vi "Test Process within Nested App Log Info Message.vi"(8 "error in (no error)":errorcluster, 11 "Test Case In":refnum<class "Logger Test.lvclass">) -> (0 "error out":errorcluster, 3 "Test Case Out":refnum<class "Logger Test.lvclass">)   [LabVIEW 2020, in "Logger Test.lvclass"]
uses:
  Logger Test.lvclass
  C:/Program Files (x86)/National Instruments/LabVIEW 2020/vi.lib/Astemes/LUnit/Test Case.lvclass
  source/Framework Test Suite/Mock Log Handler/Mock Log Handler.lvclass
  C:/Git/astemes-triarc-framework/source/Framework/Logging/Logging.lvclass
  source/Framework Test Suite/Mock Process/Mock Process.lvclass
  C:/Git/astemes-triarc-framework/source/Framework/Process/Process.lvclass
  source/Framework/Application/Application.lvclass
  source/Framework/Process/Process.lvclass/Process.ctl
  source/Framework/Application/Application.lvclass/Application.ctl
  <vilib>/Astemes/LUnit/Test Case.lvclass/Test Case.ctl
  <vilib>/Astemes/LUnit/LUnit Assertion Result.lvclass/LUnit Assertion Result.ctl
  <vilib>/Astemes/LUnit/LUnit Test Case Result.lvclass/LUnit Test Case Result.ctl
  <vilib>/Astemes/LUnit/LUnit Method Result.lvclass/LUnit Method Result.ctl
  9c4a66fc-af29-4a58-8a71-606aefca4567.vi
  ff660fc9-a87e-4241-bf4f-74109907e361.vi
  4b535133-13cd-4873-93c4-223ebd3dba1f.vi
  source/Framework/Application/Private/Add Process to Map.vi
  source/Framework/Application/Private/Start Idle Processes if Running.vi
  source/Framework/Application/Private/Throw Error If Process Already in App.vi
  source/Framework/Process/Protected/Messaging/Enqueue Message.vi
  source/Framework/Process/Public/Lifecycle/Get Lifecycle State.vi
  source/Framework/Process/Protected/SubVIs/Set Context.vi
  source/Framework/Process/Private/SubVIs/Wait for finish.vi
  source/Framework/Process/Private/SubVIs/Set Lifecycle State.vi
  <vilib>/Astemes/LUnit/Palette/Pass.vi
  <vilib>/Astemes/LUnit/Palette/Fail.vi
  <vilib>/Astemes/LUnit/Compare Variants.vi
  <vilib>/Astemes/LUnit/Describe Comparison.vi
  <vilib>/Astemes/LUnit/Set Assertion Type.vi
  source/Framework/Application/Public/Get Process.vi
  source/Framework/Process/Private/SubVIs/Handle Debug Data.vi
  source/Framework/Process/Public/Lifecycle/Leave Process Loop.vi
  <vilib>/Astemes/LUnit/Add test result.vi
  <vilib>/Astemes/LUnit/LUnit Write Passed.vi
  <vilib>/Astemes/LUnit/LUnit Write Message.vi
  <vilib>/Astemes/LUnit/LUnit Write Description.vi
  <vilib>/Astemes/LUnit/Variant to string.vi
  <vilib>/Astemes/LUnit/LUnit Write Assertion Type.vi
  source/Framework/Application/Private/Retrieve Process from App.vi
  source/Framework/Application/Private/Parse Process Name.vi
  source/Framework/Application/Private/Get Process from Map.vi
  source/Framework/Logging/Log Debug.vi
  <vilib>/AdvancedString/1D String Array to Delimited String.vi
  <vilib>/Utility/High Resolution Relative Seconds.vi
  <vilib>/Astemes/LUnit/LUnit Record Assertion Result.vi
  source/Framework/Process/Protected/Messaging/Request Message.vi
  <vilib>/AdvancedString/Delimited String to 1D String Array.vi
  <vilib>/Astemes/LUnit/LUnit Aggregate Assertion Results.vi
  source/Framework/Process/Private/SubVIs/Enqueue Request Message.vi
  <vilib>/Astemes/LUnit/Assertion Result/LUnit Read Status.vi
  <vilib>/Astemes/LUnit/LUnit Read Message.vi
  <vilib>/Astemes/LUnit/LUnit Read Description.vi
  <vilib>/Astemes/LUnit/Method Result/LUnit Merge Status.vi
  <vilib>/Astemes/LUnit/LUnit Concatenate result strings.vi
  <vilib>/Utility/error.llb/Error Cluster From Error Code.vi
  source/Framework/Process/Public/Read Name.vi
  source/Framework/Process/Private/SubVIs/Wait for Response Message.vi
  <vilib>/Utility/Data Type/Get Type Information.vi
  <vilib>/Utility/LVClass/Get LV Class Name.vi
  source/Framework/Process/Process.lvclass
  <vilib>/Astemes/LUnit/LUnit Assertion Result.lvclass
  source/Framework/Logging/Logging.lvclass
  source/Framework Test Suite/Support/Test Support.lvlib
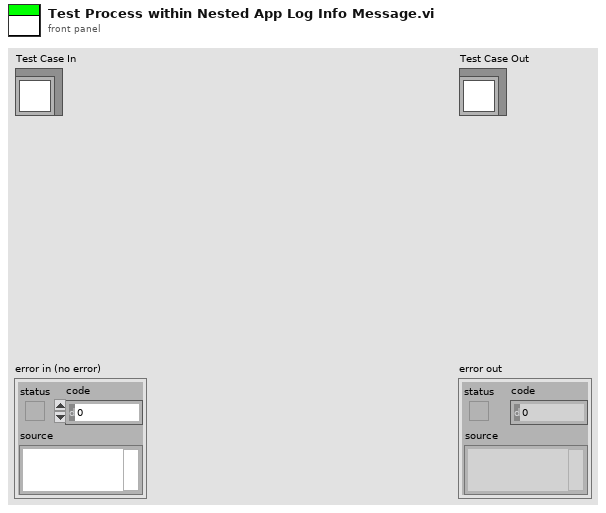
[diagram p1: front panel]
types:
  T1 = typedef "Mock Log Handler.lvclass/Log Entry.ctl" = cluster{"Level":string, "Source":string, "Message":string}
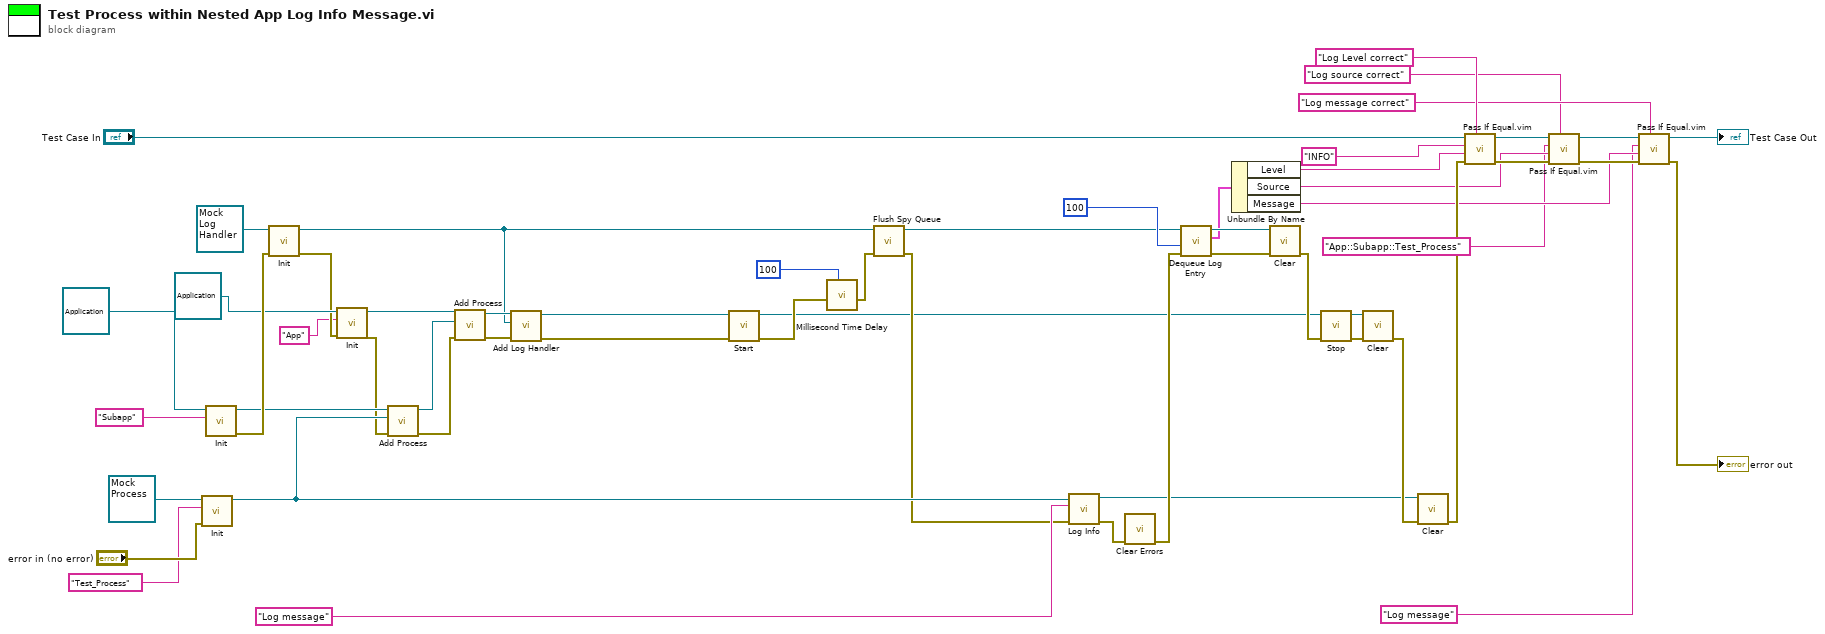
[diagram p0: block diagram]
diagram:
  n1 = call-dynamic "Init.vi"("error in (no error)"="error in (no error)", "Name"="Test_Process", "Mock Process In"=refnum<class "Mock Process.lvclass"> refnum) -> ("Mock Process Out"=w17:refnum<class "Mock Process.lvclass">)  [unwired: 7 in, 1 out]
  n2 = call-dynamic "Init.vi"("Name"="Subapp", "Process In"=refnum<class "Application.lvclass"> refnum ("Application.lvclass")) -> ("error out"=w51:errorcluster, "Process Out"=w9:refnum<class "Application.lvclass">)  [unwired: 8 in]
  n3 = call-dynamic "Init.vi"("error in (no error)"=w51, "Mock Log Handler In"=refnum<class "Mock Log Handler.lvclass"> refnum ("Mock Log Handler.lvclass")) -> ("error out"=w14:errorcluster, "Mock Log Handler Out"=w10:refnum<class "Mock Log Handler.lvclass">)  [unwired: 8 in]
  n4 = call-dynamic "Init.vi"("error in (no error)"=w14, "Name"="App", "Process In"=refnum<class "Application.lvclass"> refnum ("Application.lvclass")) -> ("error out"=w7:errorcluster, "Process Out"=w13:refnum<class "Application.lvclass">)  [unwired: 7 in]
  n5 = call "Add Process.vi"("error in (no error)"=w7, "Process"=w17, "Application In"=w9) -> ("error out"=w6:errorcluster, "Application Out"=w8:refnum<class "Application.lvclass">)  [unwired: 7 in]
  n6 = call "Add Process.vi"("error in (no error)"=w6, "Process"=w8, "Application In"=w13) -> ("error out"=w11:errorcluster, "Application Out"=w12:refnum<class "Application.lvclass">)  [unwired: 7 in]
  n7 = call "Add Log Handler.vi"("error in (no error)"=w11, "Log Handler"=w10, "Process In"=w12) -> ("error out"=w5:errorcluster, "Process Out"=w3:refnum<class "Application.lvclass">)  [unwired: 7 in]
  n8 = call "Start.vi"("error in (no error)"=w5, "Process In"=w3) -> ("error out"=w4:errorcluster, "Process Out"=w2:refnum<class "Application.lvclass">)  [unwired: 7 in, 1 out]
  n9 = call "Millisecond Time Delay.vi"("milliseconds to wait"=u32 100, "error in (no error)"=w4) -> ("error out"=w19:errorcluster)  [unwired: 7 in]
  n10 = call "Flush Spy Queue.vi"("error in (no error)"=w19, "Mock Log Handler in"=w10) -> ("error out"=w16:errorcluster, "Mock Log Handler out"=w20:refnum<class "Mock Log Handler.lvclass">)  [unwired: 7 in, 1 out]
  n11 = call "Log Info.vi"("error in (no error)"=w16, "Message"="Log message", "Logging In"=w17) -> ("error out"=w32:errorcluster, "Logging Out"=w22:refnum<class "Mock Process.lvclass">)  [unwired: 7 in]
  n12 = call <vilib>:"Clear Errors.vi"("error in (no error)"=w32) -> ("error out"=w31:errorcluster)  [unwired: 5 in, 1 out]
  n13 = call "Dequeue Log Entry.vi"("error in (no error)"=w31, "timeout in ms (-1)"=100, "Mock Log Handler in"=w20) -> ("error out"=w49:errorcluster, "Entry"=w46:T1, "Mock Log Handler out"=w50:refnum<class "Mock Log Handler.lvclass">)  [unwired: 5 in, 1 out]
  n14 = Unbundle By Name(w46) -> ("Level"=w45:string, "Source"=w35:string, "Message"=w34:string)
  n15 = call-dynamic "Clear.vi"("error in (no error)"=w49, "Mock Log Handler In"=w50) -> ("error out"=w47:errorcluster)  [unwired: 9 in]
  n16 = call "Stop.vi"("error in (no error)"=w47, "Process In"=w2) -> ("error out"=w24:errorcluster, "Process Out"=w23:refnum<class "Application.lvclass">)  [unwired: 7 in, 1 out]
  n17 = call-dynamic "Clear.vi"("error in (no error)"=w24, "Application In"=w23) -> ("error out"=w53:errorcluster)  [unwired: 9 in]
  n18 = call-dynamic "Clear.vi"("error in (no error)"=w53, "Mock Process In"=w22) -> ("error out"=w39:errorcluster)  [unwired: 9 in]
  n19 = call "Pass If Equal.vim"("Description"="Log Level correct", "error in (no error)"=w39, "Actual"=w45, "Expected"="INFO", "LUnit Test Case In"="Test Case In") -> ("error out"=w41:errorcluster, "LUnit Test Case Out"=w55:refnum<class "Logger Test.lvclass">)  [unwired: 5 in]
  n20 = call "Pass If Equal.vim"("Description"="Log source correct", "error in (no error)"=w41, "Actual"=w35, "Expected"="App::Subapp::Test_Process" ("Name"), "LUnit Test Case In"=w55) -> ("error out"=w40:errorcluster, "LUnit Test Case Out"=w43:refnum<class "Logger Test.lvclass">)  [unwired: 5 in]
  n21 = call "Pass If Equal.vim"("Description"="Log message correct", "error in (no error)"=w40, "Actual"=w34, "Expected"="Log message" ("Message"), "LUnit Test Case In"=w43) -> ("error out"=→"error out":errorcluster, "LUnit Test Case Out"=→"Test Case Out":refnum<class "Logger Test.lvclass">)  [unwired: 5 in]
